vi "Base Spectrum.vi"(8 "error in (no error)":errorcluster, 9 "Depth":u32=50, 10 "Window Width":u32=10, 11 "Spectral Processing in":refnum<class "Spectral Processing.lvclass">) -> (0 "error out":errorcluster, 3 "Spectral Processing out":refnum<class "Spectral Processing.lvclass">)   [LabVIEW 2014, in "Spectral Processing.lvclass"]
uses:
  Spectral Processing.lvclass
  <vilib>/Analysis/3filter.llb/Filter Passband Type.ctl
  Spectral Processing.lvclass/Spectral Processing.ctl
  <vilib>/Analysis/4window.llb/Gaussian Window (DBL).vi
  <vilib>/Analysis/baseanly.llb/Quick Scale 1D.vi
  <vilib>/Analysis/2dsp.llb/Inverse Real FFT.vi
  <vilib>/Analysis/3filter.llb/IIR Filter (DBL).vi
  <vilib>/Analysis/3filter.llb/Butterworth Filter (DBL).vi
  <vilib>/Analysis/3filter.llb/Zero Phase Filter (DBL).vi
  <vilib>/Analysis/NI_AALBase.lvlib
  <vilib>/Analysis/NI_AALPro.lvlib
panel:
  in  "standard deviation":dbl=0.2
  out "Processed Spectrum":dbl[][](graph)
  out "Fourier Domain":dbl[][](graph)
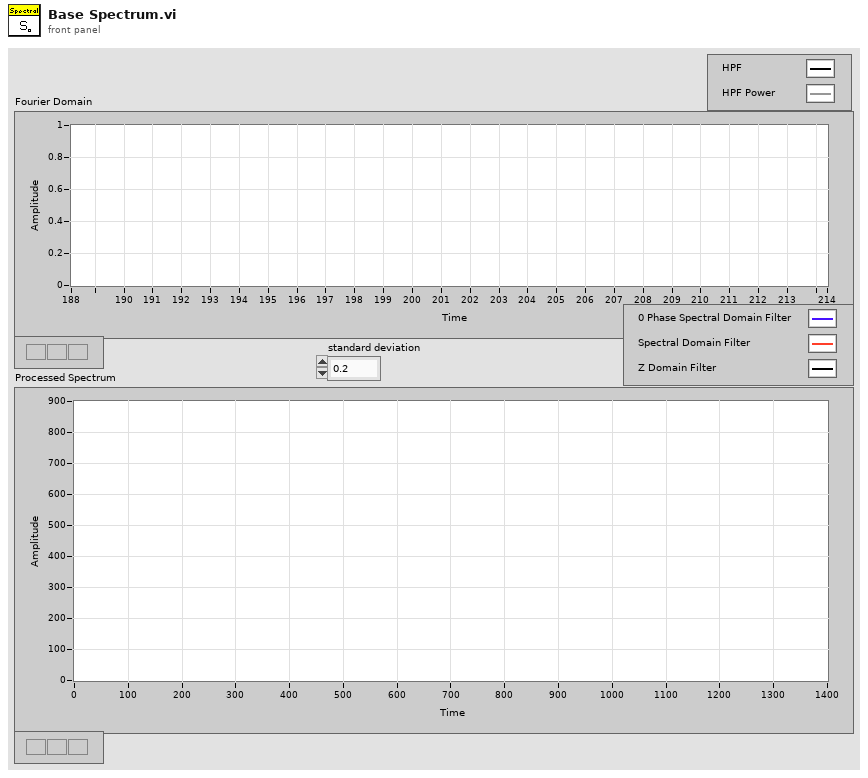
[diagram p1: front panel]
types:
  T1 = typedef "NI_AALBase.lvlib/Filter Passband Type.ctl" = enum32{"Lowpass", "Highpass", "Bandpass", "Bandstop"}
  T2 = cluster{"filter structure":enum32{"IIR 2nd Order", "IIR 4th Order"}, "Reverse Coefficients":dbl[], "Forward Coefficients":dbl[]}
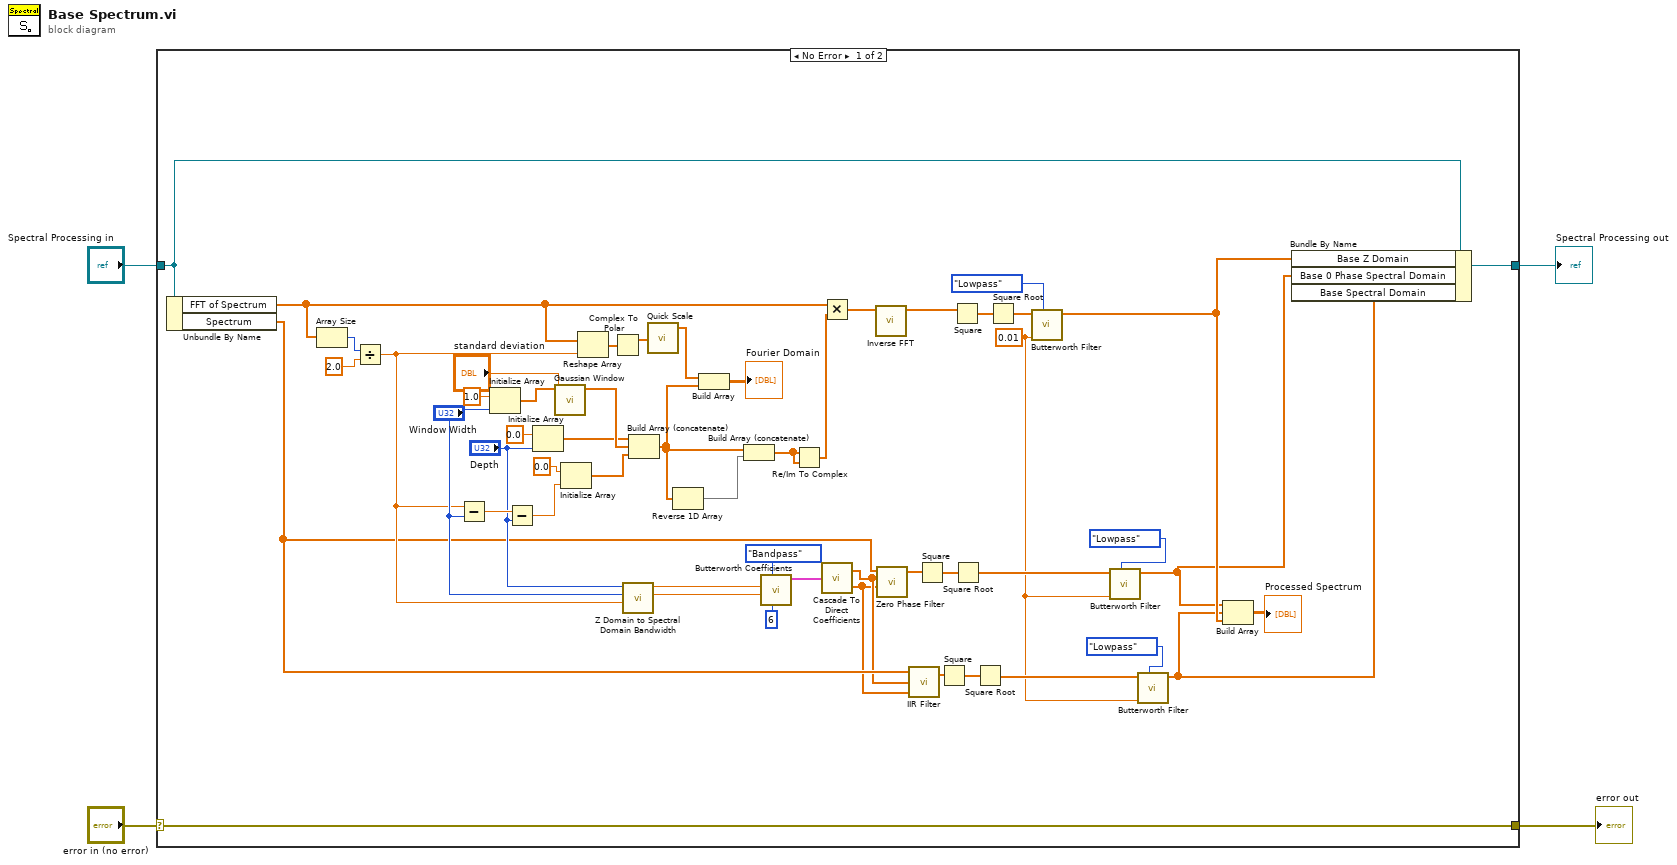
[diagram p0: block diagram]
diagram:
  n1 = case shown="No Error" "error in (no error)" {
    selector: "error in (no error)" -> [w57 w59]
    tunnel: [w57 w59] -> w3
    tunnel: [w10 w58] -> w1
    tunnel: "Spectral Processing in" -> [w9 w58]
    frame No Error {
      w14 = 0.01 ("low cutoff freq: fl")
      n2 = Unbundle By Name(w9) -> ("FFT of Spectrum"=w44:cdb[], "Spectrum"=w24:dbl[])
      n3 = Array Size(array=w44) -> (size(s)=w30:i32)
      n4 = Divide(x=w30, y=2.0 ("element")) -> (x/y=w26:dbl)
      n5 = Subtract(x=w26, y="Window Width") -> (x-y=w52:dbl)
      n6 = Initialize Array(1.0 ("element"), "Window Width") -> (w56:dbl[])
      n7 = Subtract(x=w52, y="Depth") -> (x-y=w51:dbl)
      n8 = Initialize Array(0.0 ("element"), "Depth") -> (w49:dbl[])
      n9 = call-poly <vilib>:"Gaussian Window.vi"("standard deviation"="standard deviation", "X"=w56) -> ("Windowed X"=w50:dbl[])  [unwired: 8 in, 1 out]
      n10 = Initialize Array(0.0 ("element"), w51) -> (w48:dbl[])
      n11 = Reshape Array(w44, w26) -> (w43:cdb[])
      n12 = Complex To Polar(r * e^(i*theta)=w43) -> (r=w42:dbl[])  [unwired: 1 out]
      n13 = call "Z Domain to Spectral Domain Bandwidth.vi"("Samples"=w26, "Window Width"="Window Width", "Depth"="Depth") -> ("Low Pass Freq (scaled)"=w27:dbl, "High Pass Freq (Scaled)"=w28:dbl)  [unwired: 7 in]
      n14 = Build Array (concatenate)(w49, w50, w48) -> (w45:dbl[])
      n15 = call-poly <vilib>:"Quick Scale.vi"("X"=w42) -> ("Y[i]=X[i]/Max|X|"=w41:dbl[])  [unwired: 2 out]
      n16 = Reverse 1D Array(array=w45) -> (reversed array=w46:dbl[])
      n17 = Build Array(w41, w45) -> (→"Fourier Domain":dbl[][])
      n18 = Build Array (concatenate)(w45, w46) -> (w25:dbl[])
      n19 = call <vilib>:"Butterworth Coefficients.vi"("order"=6, "filter type"=Filter_Passband_Type."Bandpass", "low cutoff freq: fl"=w27, "high cutoff freq: fh"=w28) -> ("IIR Filter Cluster"=w40:T2)  [unwired: 6 in, 1 out]
      n20 = Re/Im To Complex(1:w25, 2:w25) -> (0:w13:cdb[])
      n21 = Multiply(x=w44, y=w13) -> (x*y=w12:cdb[])
      n22 = call <vilib>:"Cascade To Direct Coefficients.vi"("IIR Filter Cluster"=w40) -> ("Reverse Coefficients"=w22:dbl[], "Forward Coefficients"=w21:dbl[])
      n23 = call-poly <vilib>:"Inverse FFT.vi"("FFT {X}"=w12) -> ("X"=w34:dbl[])  [unwired: 9 in, 1 out]
      n24 = call-poly <vilib>:"Zero Phase Filter.vi"("Forward Coefficients"=w21, "Reverse Coefficients"=w22, "X"=w24) -> ("Filtered X"=w37:dbl[])  [unwired: 7 in, 1 out]
      n25 = call-poly <vilib>:"IIR Filter.vi"("Forward Coefficients"=w21, "Reverse Coefficients"=w22, "X"=w24) -> ("Filtered X"=w23:dbl[])  [unwired: 1 in, 1 out]
      n26 = Square(x=w37) -> (x^2=w36:dbl[])
      n27 = Square(x=w23) -> (x^2=w29:dbl[])
      n28 = Square(x=w34) -> (x^2=w35:dbl[])
      n29 = Square Root(x=w36) -> (sqrt(x)=w19:dbl[])
      n30 = Square Root(x=w29) -> (sqrt(x)=w20:dbl[])
      n31 = Square Root(x=w35) -> (sqrt(x)=w18:dbl[])
      n32 = call-poly <vilib>:"Butterworth Filter.vi"("filter type"=Filter_Passband_Type."Lowpass", "low cutoff freq: fl"=w14, "X"=w18) -> ("Filtered X"=w8:dbl[])  [unwired: 5 in, 1 out]
      n33 = call-poly <vilib>:"Butterworth Filter.vi"("filter type"=Filter_Passband_Type."Lowpass", "low cutoff freq: fl"=w14, "X"=w19) -> ("Filtered X"=w7:dbl[])  [unwired: 5 in, 1 out]
      n34 = call-poly <vilib>:"Butterworth Filter.vi"("filter type"=Filter_Passband_Type."Lowpass", "low cutoff freq: fl"=w14, "X"=w20) -> ("Filtered X"=w6:dbl[])  [unwired: 5 in, 1 out]
      n35 = Build Array(w7, w6, w8) -> (→"Processed Spectrum":dbl[][])
      n36 = Bundle By Name(cluster=w9, "Base Z Domain"=w8, "Base 0 Phase Spectral Domain"=w7, "Base Spectral Domain"=w6) -> (w10:refnum<class "Spectral Processing.lvclass">)
    }
    frame Error {
    }
  }
  "error out" <- w3
  "Spectral Processing out" <- w1
